vi "Grab and Broadcast (Listener).vi"() -> ()   [LabVIEW 2011]
doc: "The Grab and Broadcast (Listener) VI acquires images continuously and displays the images in an image control using high-level acquisition VIs. This VI also demonstrates how to acquire data from a shared camera in a broadcasting application. A grab is appropriate for high-speed applications in which you need to process only one image at a time."
uses:
  <vilib>/vision/driver/NI_Vision_Acquisition_Software.lvlib
  <vilib>/vision/driver/IMAQdx.llb/IMAQdx Camera Control Mode.ctl
panel:
  in  "Camera Name":refnum<k21> caption="IMAQdx Session"
  out "Buffer Number":u32
  out "Image":T1(plugin-control)
  out "Frame Rate":dbl(knob) scale=0.0..100.0
  in  "Stop":bool
  # "Overview: Demonstrates how to acquire images that are broadcast from a controller so multiple machines can acquire the same images from a camera.\nRequirements: Vision Acquisition Software\nInstructions: \n1. Select the Camera Name. \n2. Run the Grab and Broadcast (Controller) VI on a different machine or target. Make sure the Camera Name references the same camera in both examples.  \n3. Run the Grab and Broadcast (Listener) VI."
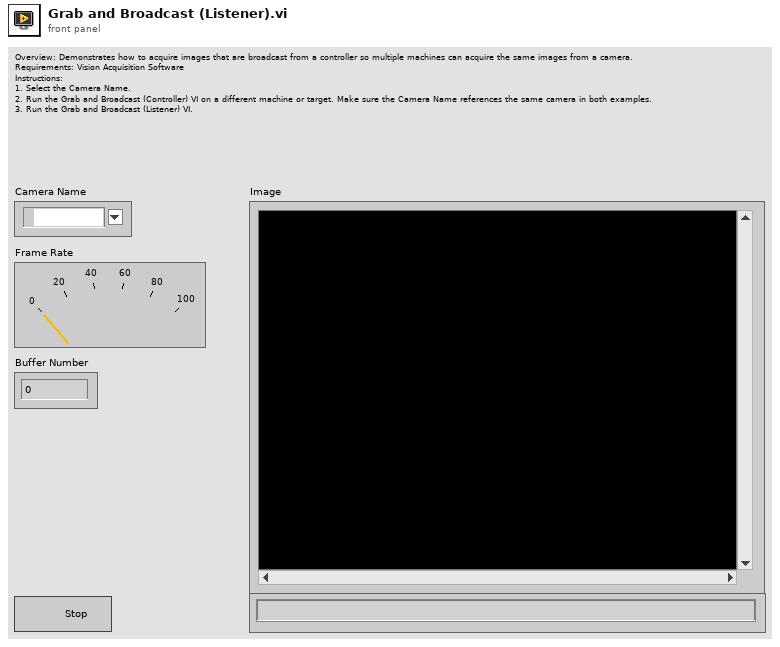
[diagram p1: front panel]
types:
  T1 = typedef "IMAQ Image.ctl" = refnum<image>
  T2 = typedef "NI_Vision_Acquisition_Software.lvlib/IMAQdx Camera Control Mode.ctl" = enum32{"Controller", "Listener"}
  T3 = typedef "IMAQdx.ctl" = refnum<k21>
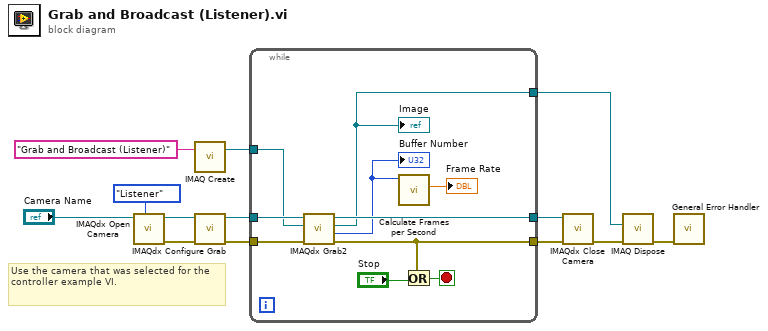
[diagram p0: block diagram]
diagram:
  # "Use the camera that was selected for the controller example VI."
  n1 = call <vilib>:"IMAQdx Open Camera.vi"("Camera Control Mode"=IMAQdx_Camera_Control_Mode."Listener", "Session In"="Camera Name") -> ("error out"=w8:errorcluster, "Session Out"=w7:T3)  [unwired: 1 in, 7 out]
  n2 = call "IMAQ Create"("Image Name"="Grab and Broadcast (Listener)") -> ("New Image"=w13:T1)  [unwired: 3 in, 2 out]
  n3 = call <vilib>:"IMAQdx Configure Grab.vi"("error in"=w8, "Session In"=w7) -> ("error out"=w11:errorcluster, "Session Out"=w12:T3)  [unwired: 8 out]
  n4 = while {
    tunnel: [w18] -> w10
    tunnel: w11 -> [w20]
    tunnel: w12 -> [w21]
    tunnel: [w15] -> w9
    tunnel: w13 -> [w19]
    tunnel: [w14] -> w5
    stop <- w23 stop-if-true
    n5 = call <vilib>:"IMAQdx Grab2.vi"("error in"=w20, "Image In"=w19, "Session In"=w21) -> ("error out"=w15:errorcluster, "Buffer Number Out"=w16:u32, "Image Out"=w14:T1, "Session Out"=w18:T3)  [unwired: 5 in]
    "Image" <- w14
    "Buffer Number" <- w16
    n6 = call <vilib>:"Calculate Frames per Second.vi"("Buffer Number"=w16) -> ("Processed Frames/s"=→"Frame Rate":dbl)  [unwired: 8 in, 2 out]
    n7 = Or(x=w15, y="Stop") -> (x .or. y?=w23:bool)
  }
  n8 = call <vilib>:"IMAQdx Close Camera.vi"("error in"=w9, "Session In"=w10) -> ("error out"=w4:errorcluster)  [unwired: 9 out]
  n9 = call "IMAQ Dispose"("Image"=w5, "error in (no error)"=w4) -> ("error out"=w3:errorcluster)  [unwired: 4 in]
  n10 = call <vilib>:"General Error Handler.vi"("error in (no error)"=w3) -> ()  [unwired: 1 in, 14 out]
